vi "okCFrontPanelDevices Destroy Device Refnum.vi"(8 "error in (no error)":errorcluster, 11 "okCFrontPanel Device Refnum":refnum<k24>) -> (0 "error out":errorcluster)   [LabVIEW 2019, in "okFrontPanelC#Wrapper.lvlib"]
uses:
  okFrontPanelC#Wrapper.lvlib
  C:/UCLA Thinkpad Google Drive/LabVIEW 2019 SP1/builds/SS2 Live Distribution/Opal Kelly/C# Wrapper/libFrontPanel-csharp.dll
  libFrontPanel-csharp.dll
  okTDeviceInfo Struct.ctl
  okEDeviceInterface.ctl
  okTFlashLayoutStruct.ctl
  okTProductID.ctl
  okEUSBSpeed.ctl
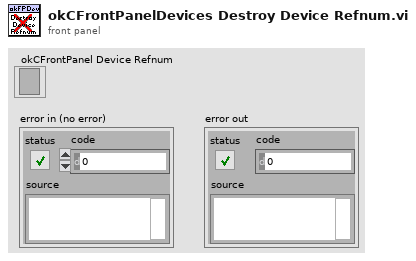
[diagram p1: front panel]
types:
  T1 = typedef "okFrontPanelC#Wrapper.lvlib/okTDeviceInfo Struct.ctl" = cluster{"deviceID":string, "okInterface":T2, "deviceMajorVersion":i32, "deviceMinorVersion":i32, "FPGA Flash Memory Layout":T3, "System Flash Memory Layout":T3, "hasFMCEEPROM":bool, "hasResetProfiles":bool, "hostInterfaceMajorVersion":i32, "hostInterfaceMinorVersion":i32, "isFrontPanelEnabled":bool, "isPLL22150Supported":bool, "isPLL22393Supported":bool, "pipeWidth":i32, "Device ID":T4, "productName":string, "registerAddressWidth":i32, "registerDataWidth":i32, "serialNumber":string, "triggerWidth":i32, "USB Speed":T5, "wireWidth":i32}
  T2 = typedef "okFrontPanelC#Wrapper.lvlib/okEDeviceInterface.ctl" = enum16{"unknown", "USB2", "PCIe", "USB3"}
  T3 = typedef "okFrontPanelC#Wrapper.lvlib/okTFlashLayoutStruct.ctl" = cluster{"maxUserSector":u32, "minUserSector":u32, "pageSize":u32, "sectorCount":u32, "sectorSize":u32}
  T4 = typedef "okFrontPanelC#Wrapper.lvlib/okTProductID.ctl" = enum16{"UNKNOWN", "XEM3001V1", "XEM3001V2", "XEM3010", "XEM3005", "XEM3001CL", "XEM3020", "XEM3050", "XEM9002", "XEM3001RB", "XEM5010", "XEM6110LX45", "XEM6001", "XEM6010LX45", "XEM6010LX150", "XEM6110LX150", "XEM6006LX9", "XEM6006LX16", "XEM6006LX25", "XEM5010LX110", "ZEM4310", "XEM6310LX45", "XEM6310LX150", "XEM6110V2LX45", "XEM6110V2LX150", "XEM6002LX9", "XEM6310MTLX45T", "XEM6320LX130T", "XEM7350K70T", "XEM7350K160T", "XEM7350K410T", "XEM6310MTLX150T", "ZEM5305A2", "ZEM5305A7", "XEM7001A15", "XEM7001A35", "XEM7360K160T", "XEM7360K410T", "ZEM5310A4", "ZEM5310A7", "ZEM5370A5", "XEM7010A50", "XEM7010A200", "XEM7310A75", "XEM7310A200", "XEM7320A75T", "XEM7320A200T", "XEM7305", "FPXBARE"}
  T5 = typedef "okFrontPanelC#Wrapper.lvlib/okEUSBSpeed.ctl" = enum16{"unknown", "Full", "High", "Super"}
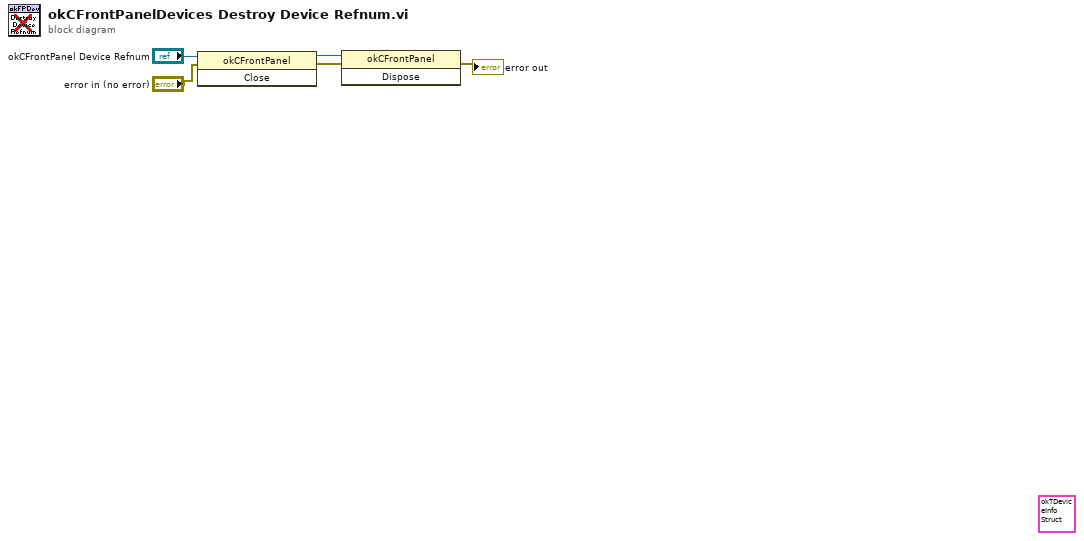
[diagram p0: block diagram]
diagram:
  (unwired) T1 {"deviceID"="", "okInterface"=enum."unknown", "deviceMajorVersion"=0, "deviceMinorVersion"=0, "FPGA Flash Memory Layout"={"maxUserSector"=0, "minUserSector"=0, "pageSize"=0, "sectorCount"=0, "sectorSize"=0}, "System Flash Memory Layout"={"maxUserSector"=0, "minUserSector"=0, "pageSize"=0, "sectorCount"=0, "sectorSize"=0}, "hasFMCEEPROM"=FALSE, "hasResetProfiles"=FALSE, "hostInterfaceMajorVersion"=0, "hostInterfaceMinorVersion"=0, "isFrontPanelEnabled"=FALSE, "isPLL22150Supported"=FALSE, "isPLL22393Supported"=FALSE, "pipeWidth"=0, "Device ID"=enum."UNKNOWN", "productName"="", "registerAddressWidth"=0, "registerDataWidth"=0, "serialNumber"="", "triggerWidth"=0, "USB Speed"=enum."unknown", "wireWidth"=0} ("Device Info")
  n1 = invoke class="okCFrontPanel" method="Close"(reference="okCFrontPanel Device Refnum", error in="error in (no error)") -> (reference out=w2:refnum<k24>, error out=w1:errorcluster)  [unwired: 1 in, 1 out]
  n2 = invoke class="okCFrontPanel" method="Dispose"(reference=w2, error in=w1) -> (error out=→"error out":errorcluster)  [unwired: 1 in, 2 out]
